vi "build.procElement.vi"(11 "UiBuildProcHead":T1={"Procedure Name"="MyProcExample", "Running"=TRUE, "tags"="MyProcExample"}) -> (0 "error out":errorcluster, 3 "procElement out":variant)   [LabVIEW 2024]
uses:
  controls/UiProcHeader.ctl
  controls/typeProcVarientName.ctl
  Polymorphics/variantCtrlString.vi
  Polymorphics/variantCtrlBoolean.vi
  Polymorphics/variantCtrlNumber.vi
  proc.util.validateParamExist.vi
  <vilib>/Utility/error.llb/Clear Errors.vi
  util.error.create.vi
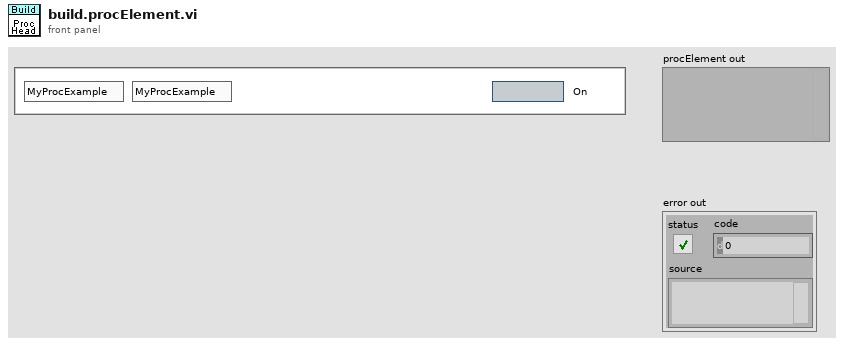
[diagram p1: front panel]
types:
  T1 = typedef "UiProcHeader.ctl" = cluster{"Procedure Name":string, "Running":bool, "tags":string}
  T2 = typedef "typeProcVarientName.ctl" = enum16{"procNameID", "procModuleID", "procPath", "procIsRunning", "procIndex", "procModule", "procRegisterNumeric", "procRegisterString", "procReport", "procReportPrev", "procCLK", "procStepPointer", "procType"}
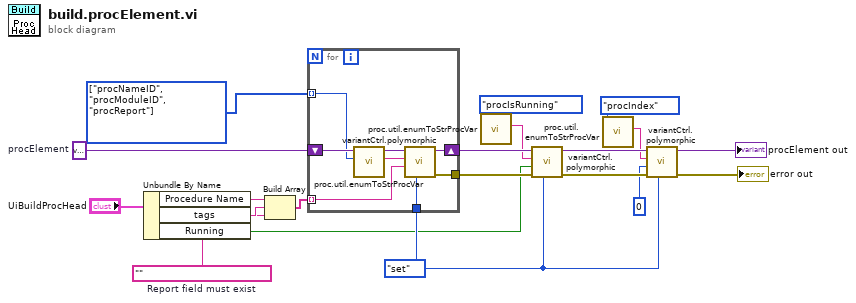
[diagram p0: block diagram]
diagram:
  w2 = ""  # Report field must exist
  w6 = enum16{"get", "set"}."set" ("menu in (get)")
  w18 = T2[] [enum."procNameID", enum."procModuleID", enum."procReport"] items=["procNameID", "procModuleID", "procPath", "procIsRunning", "procIndex", "procModule", "procRegisterNumeric", "procRegisterString", "procReport", "procReportPrev", "procCLK", "procStepPointer", "procType"] ("Proc var")
  w20 = variant  # procElement
  n1 = Unbundle By Name("UiBuildProcHead") -> ("Procedure Name"=w12:string, "tags"=w3:string, "Running"=w5:bool)
  n2 = Build Array(w12, w3, w2) -> (w4:string[])
  n3 = for {
    tunnel: w18 -> [w26] mode=indexing
    tunnel: [w23] -> w14
    tunnel: w4 -> [w22] mode=indexing
    tunnel: w6 -> [w21]
    shift-right: [w24] -> w17
    shift-left: w20 -> [w27]
    n4 = call "proc.util.enumToStrProcVar.vi"("Proc var"=w26) -> ("String"=w25:string)  [unwired: 10 in]
    n5 = call-poly "variantCtrl.polymorphic.vi"("menu in (get)"=w21, "String Value"=w22, "name in"=w25, "Step in"=w27) -> ("error out"=w23:errorcluster, "Step out"=w24:variant)  [unwired: 4 in, 2 out]
  }
  n6 = call "proc.util.enumToStrProcVar.vi"("Proc var"=typeProcVarientName."procIsRunning") -> ("String"=w15:string)  [unwired: 10 in]
  n7 = call-poly "variantCtrl.polymorphic.vi"("menu in (get)"=w6, "error in"=w14, "Boolean Value in"=w5, "name in"=w15, "variant in"=w17) -> ("error out"=w11:errorcluster, "variant out"=w19:variant)  [unwired: 3 in, 2 out]
  n8 = call "proc.util.enumToStrProcVar.vi"("Proc var"=typeProcVarientName."procIndex") -> ("String"=w9:string)  [unwired: 10 in]
  n9 = call-poly "variantCtrl.polymorphic.vi"("menu in (get)"=w6, "error in"=w11, "number"=0, "name in"=w9, "variant in"=w19) -> ("error out"=→"error out":errorcluster, "variant out"=→"procElement out":variant)  [unwired: 3 in, 2 out]
